vi "005TimeToGroundAns.vi"() -> ()   [LabVIEW 2010]
panel:
  in  "g":dbl
  out "timeToHitGround [s]":dbl
  in  "height [meters from ground]":dbl
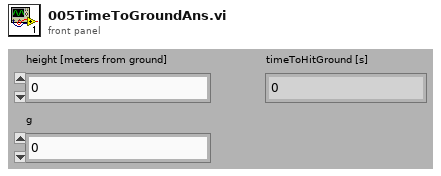
[diagram p1: front panel]
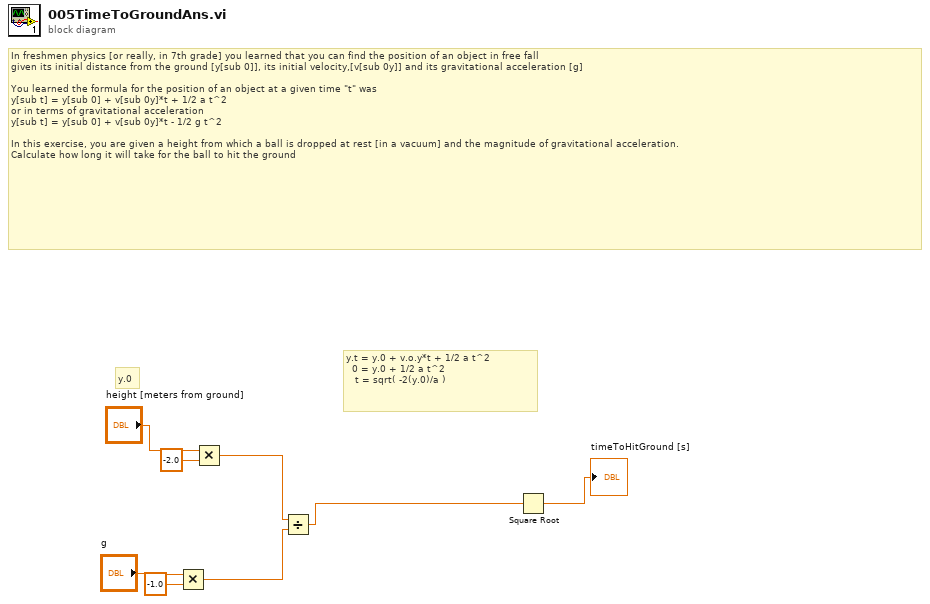
[diagram p0: block diagram]
diagram:
  # "y.0"
  # "y.t = y.0 + v.o.y*t + 1/2 a t^2\n  0 = y.0 + 1/2 a t^2\n   t = sqrt( -2(y.0)/a )"
  # "In freshmen physics [or really, in 7th grade] you learned that you can find the position of an object in free fall\ngiven its initial distance from the ground [y[sub 0]], its initial velocity,[v[sub 0y]] and its gravitational acceleration [g]\n\nYou learned the formula for the position of an object at a given time \"t\" was\ny[sub t] = y[sub 0] + v[sub 0y]*t + 1/2 a t^2\nor in terms of gravitational acceleration\ny[sub t] = y[sub 0] + v[sub 0y]*t - 1/2 g t^2\n\nIn this exercise, you are given a height from which a ball is dropped at rest [in a vacuum] and the magnitude of gravitational acceleration.\nCalculate how long it will take for the ball to hit the ground"
  n1 = Multiply(x="g", y=-1.0) -> (x*y=w6:dbl)
  n2 = Multiply(x="height [meters from ground]", y=-2.0) -> (x*y=w3:dbl)
  n3 = Divide(x=w3, y=w6) -> (x/y=w2:dbl)
  n4 = Square Root(x=w2) -> (sqrt(x)=→"timeToHitGround [s]":dbl)
